vi "Ke2400 Test.vi"() -> ()   [LabVIEW 2012]
panel:
  out "Voltage(V)":string
  out "error out":errorcluster
  out "uA":string
  in  "Volt Level":dbl
  in  "Idd Compliace(mA)":dbl=6.0
  in  "error in (no error)":errorcluster
  in  "VISA resource name":refnum<visa-resource-name>
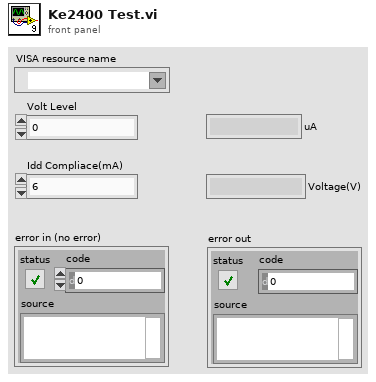
[diagram p1: front panel]
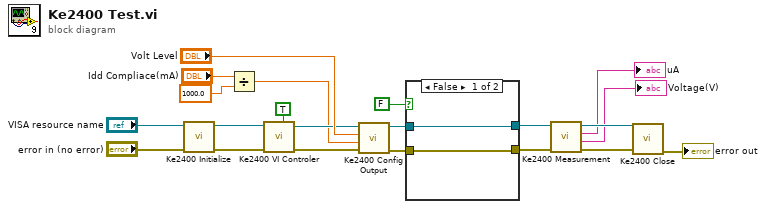
[diagram p0: block diagram]
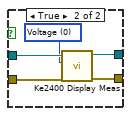
[diagram p2: hidden frame]
diagram:
  n1 = call "Ke2400 Initialize.vi"("error in (no error)"="error in (no error)", "VISA resource name"="VISA resource name") -> ("error out"=w20:errorcluster, "VISA resource name out"=w21:refnum<visa-resource-name>)  [unwired: 8 in]
  n2 = Divide(x="Idd Compliace(mA)", y=1000.0) -> (x/y=w2:dbl)
  n3 = call "Ke2400 VI Controler.vi"("ON/OFF"=TRUE, "error in (no error)"=w20, "VISA In"=w21) -> ("error out"=w16:errorcluster, "VISA Out"=w14:refnum<visa-resource-name>)  [unwired: 7 in]
  n4 = call "Ke2400 Config Output.vi"("error in (no error)"=w16, "Compliance  Level (0.1)"=w2, "Output Level (0)"="Volt Level", "VISA resource name"=w14) -> ("error out"=w11:errorcluster, "VISA resource name out"=w12:refnum<visa-resource-name>)  [unwired: 6 in]
  n5 = case shown="False" FALSE {
    tunnel: w12 -> [w23 w28]
    tunnel: w11 -> [w22 w27]
    tunnel: [w22 w25] -> w10
    tunnel: [w23 w24] -> w9
    frame False {
    }
    frame True {
      w26 = u16 0 items=["Voltage", "Current", "Resistance"] ("Display Measurement")
      n6 = call "Ke2400 Display Meas.vi"("error in (no error)"=w27, "Display Measurement"=w26, "VISA resource name"=w28) -> ("error out"=w25:errorcluster, "VISA resource name out"=w24:refnum<visa-resource-name>)  [unwired: 7 in]
    }
  }
  n7 = call "Ke2400 Measurement.vi"("error in (no error)"=w10, "VISA in"=w9) -> ("error out"=w8:errorcluster, "Voltage(V)"=→"Voltage(V)":string, "uA"=→"uA":string, "VISA Out"=w7:refnum<visa-resource-name>)  [unwired: 6 in]
  n8 = call "Ke2400 Close.vi"("error in (no error)"=w8, "VISA resource name"=w7) -> ("error out"=→"error out":errorcluster)  [unwired: 9 in]
